vi "Select Single Control.vi"(8 "error in (no error)":errorcluster, 10 "Ctl Refnum":refnum<vi>, 11 "Editor in":refnum<class "Editor.lvclass">) -> (0 "error out":errorcluster, 3 "Editor out":refnum<class "Editor.lvclass">)   [LabVIEW 2020, in "VolatusGUIEditor.lvlib" / "Editor.lvclass"]
uses:
  Editor.lvclass
  Editor.lvclass/Editor.ctl
  Selection Mode.ctl
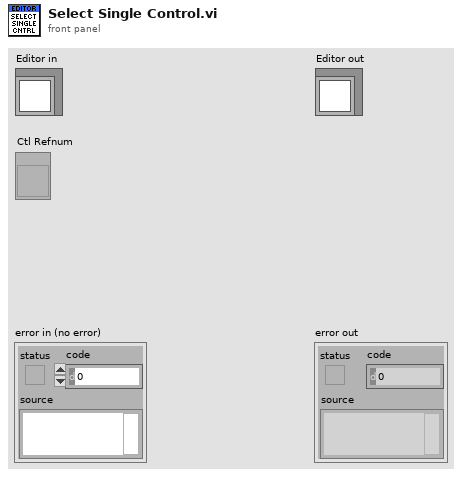
[diagram p1: front panel]
types:
  T1 = typedef "VolatusGUIEditor.lvlib/Editor.lvclass/Selection Mode.ctl" = enum16{"None", "Single", "Multi"}
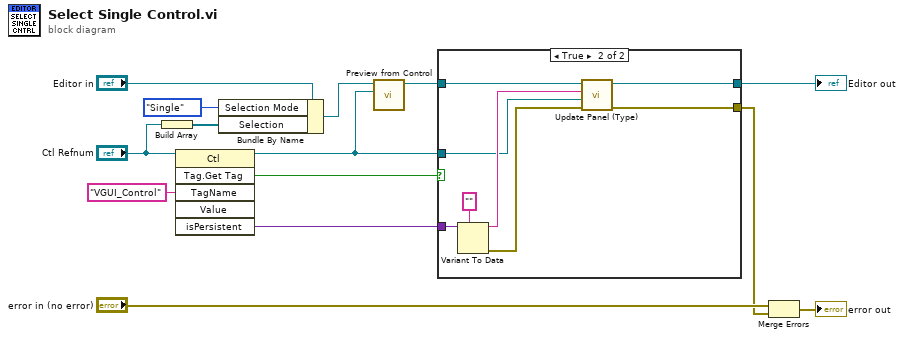
[diagram p0: block diagram]
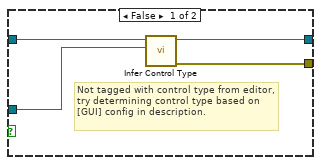
[diagram p2: hidden frame]
diagram:
  n1 = Build Array("Ctl Refnum") -> (w11:refnum<vi>[])
  n2 = invoke class="Ctl" method="Tag.Get Tag"(reference="Ctl Refnum", "TagName"="VGUI_Control" ("Tag Name")) -> (reference out=w2:refnum<vi>, "GetTag"=w7:bool, "isPersistent"=w8:variant)  [unwired: 4 in, 3 out]
  n3 = Bundle By Name(cluster="Editor in", "Selection Mode"=Selection_Mode."Single", "Selection"=w11) -> (w6:refnum<class "Editor.lvclass">)
  n4 = call "Preview from Control.vi"("Ctl Refnum"=w2, "Editor in"=w6) -> ("Editor out"=w3:refnum<class "Editor.lvclass">)  [unwired: 8 in, 1 out]
  n5 = case shown="True" w7 {
    tunnel: w8 -> [_ w26]
    tunnel: w3 -> [w18 w24]
    tunnel: [w17 w23] -> w5
    tunnel: w2 -> [w16 w19]
    tunnel: [w15 w20] -> w1
    frame False {
      # "Not tagged with control type from editor, try determining control type based on [GUI] config in description."
      n6 = call "Infer Control Type.vi"("Ctl Refnum"=w16, "Editor in"=w18) -> ("error out"=w15:errorcluster, "Editor out"=w17:refnum<class "Editor.lvclass">)  [unwired: 8 in]
    }
    frame True {
      n7 = Variant To Data(type="", Variant=w26) -> (data=w22:string, error out=w21:errorcluster)  [unwired: 1 in]
      n8 = call "Update Panel (Type).vi"("error in (no error)"=w21, "Ctl Refnum"=w19, "Control Type"=w22, "Editor in"=w24) -> ("error out"=w20:errorcluster, "Editor out"=w23:refnum<class "Editor.lvclass">)  [unwired: 6 in]
    }
  }
  "Editor out" <- w5
  n9 = Merge Errors("error in (no error)", w1) -> (→"error out":errorcluster)
